vi "PCP return string to variant.vi"(1 "Action":T1, 7 "PCP return string":string, 11 "error in (no error)":errorcluster) -> (8 "Data":variant, 15 "error out":errorcluster)   [LabVIEW 2011]
uses:
  PCP Commands.ctl
  PCP return data types/RDd return.ctl
  PCP return data types/RA return Analog I.ctl
  PCP return data types/RP return digital IO.ctl
  PCP Command definer.ctl
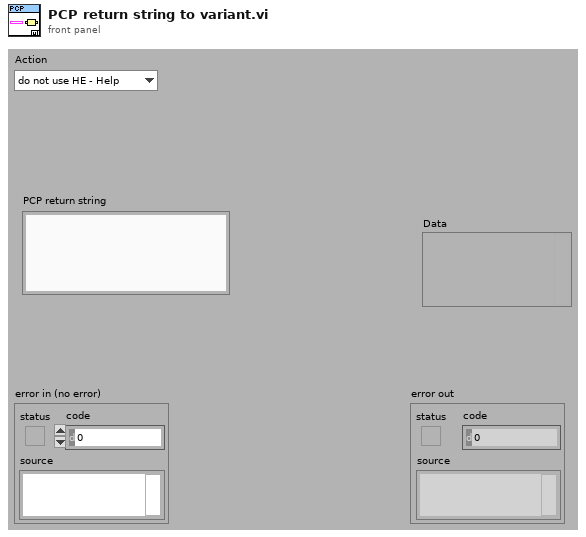
[diagram p1: front panel]
types:
  T1 = typedef "PCP Commands.ctl" = enum16{"do not use HE - Help", "RDd - Most used inputs", "RA - All analog inputs", "RE n Reset DO n", "SE n Set DO n", "RP - Get digital inputs", "VA d Set AO A  Motor Volt", "VB d Set AO B  Cable Resistance", "VEr - Get Version", "DYp - Depth counter", "DR - Reset Depth Counter", "DS n Set Depth options(0-3)", "do not use ME - Manual mode enabled", "MD - Manual mode disabled", "ID - Get ID(2001)", "TS - Get Timestamp", "TO d(s)  Set timeout", "do not use LO n Start Loop Mode(1,2)", "AL n RD&LO variation", "ST - Stop Loop Mode"}
  T2 = typedef "PCP Command definer.ctl" = cluster{"Action":T1, "n(0)":i32, "d(0.0)":dbl}
  T3 = typedef "RP return digital IO.ctl" = cluster{"DO -  HVPSU HV Off":bool, "DO -  HVPSU HV On":bool, "DI -  Unused 1":bool, "DO -  Local(T) / PC(F) mode":bool, "DI - Unused 2":bool, "DI - HVPSU HV On(T)":bool, "DI - PCP Local control(T)":bool, "DI - HVPSU On(T)":bool}
  T4 = typedef "RA return Analog I.ctl" = cluster{"HVPSU voltage output (AI 1)":dbl, "HVPSU current output (AI 2)":dbl, "PCP Motor voltage, head voltage (AI 3)":dbl, "PCP Cable resistance (AI 4)":dbl, "Cable tension (AI 5)":dbl, "CCL (AI 6)":dbl}
  T5 = typedef "RDd return.ctl" = cluster{"AI":T4, "Depth counter(Raw)":i32, "General Ratemeter":dbl, "Digital ports":T3}
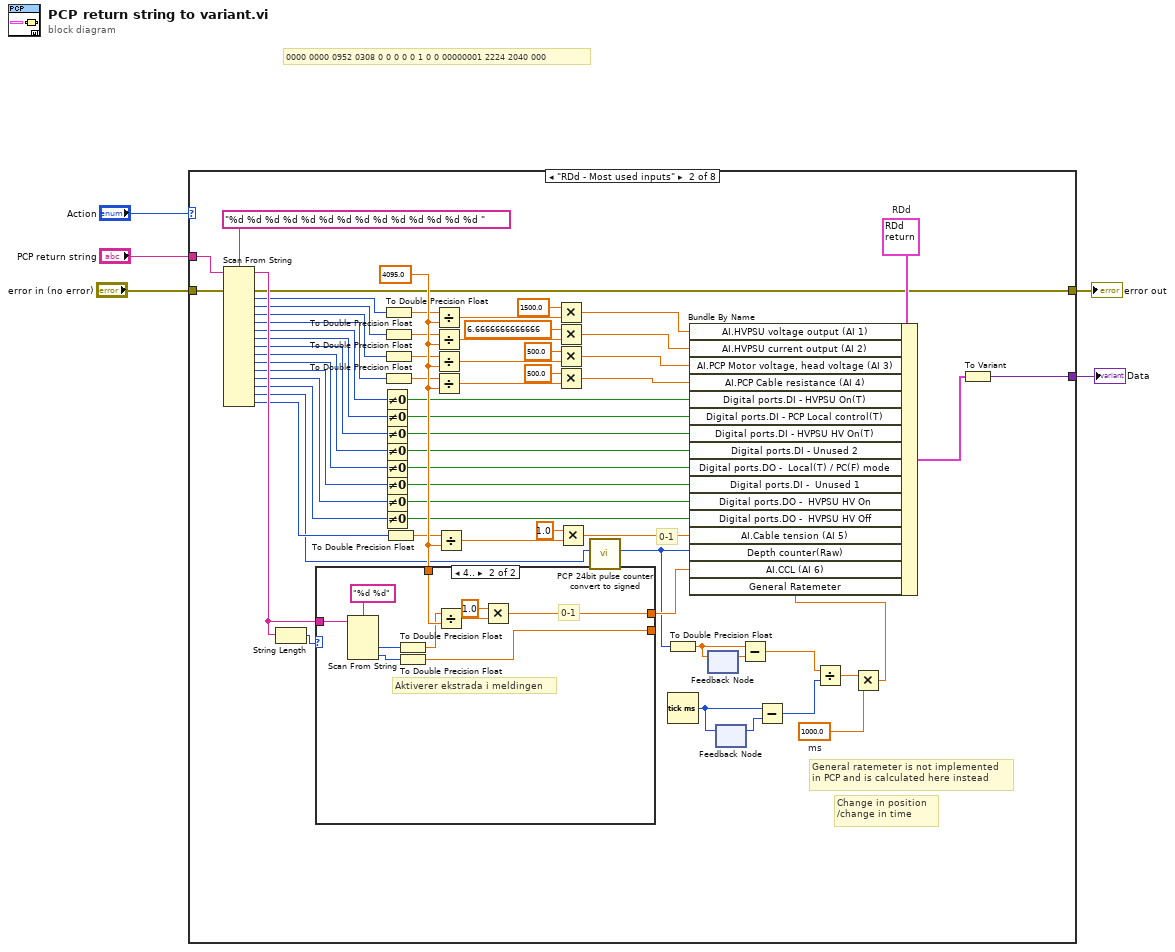
[diagram p0: block diagram]
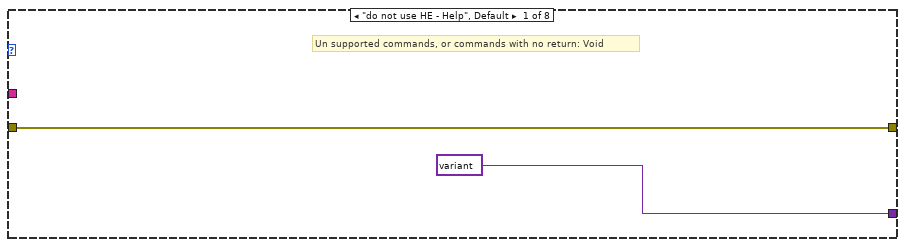
[diagram p2: hidden frame]
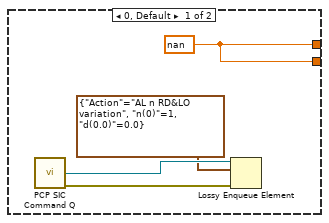
[diagram p3: hidden frame]
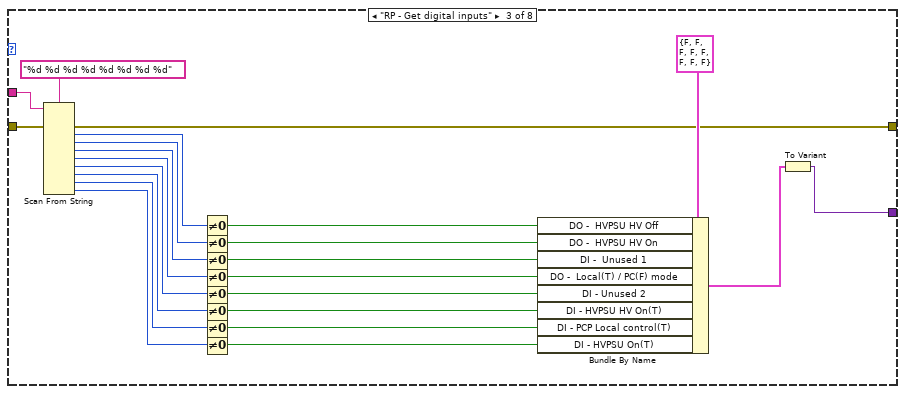
[diagram p4: hidden frame]
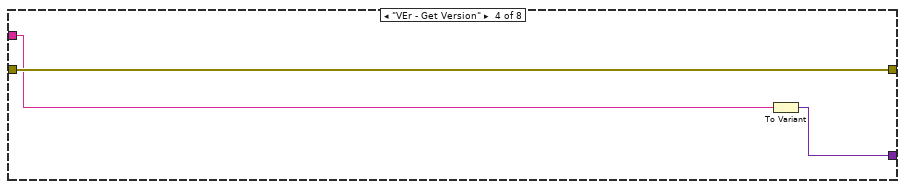
[diagram p5: hidden frame]
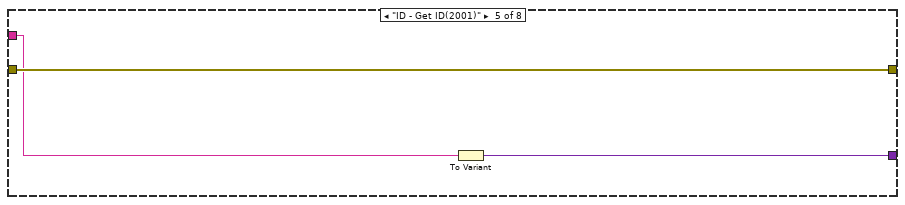
[diagram p6: hidden frame]
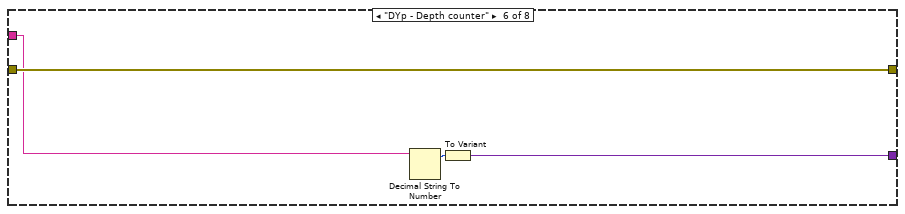
[diagram p7: hidden frame]
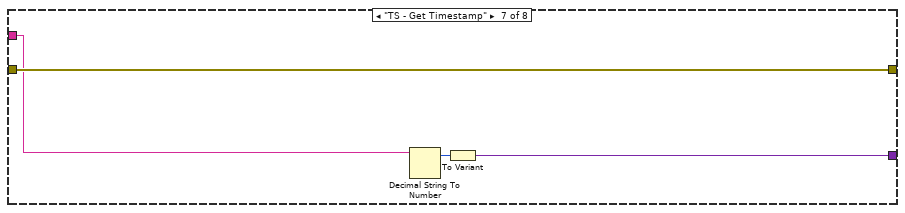
[diagram p8: hidden frame]
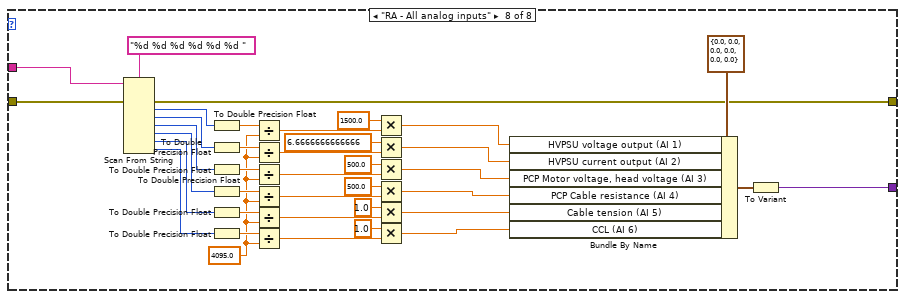
[diagram p9: hidden frame]
diagram:
  # "0000 0000 0952 0308 0 0 0 0 0 1 0 0 00000001 2224 2040 000"
  n1 = case shown="\"RDd - Most used inputs\"" "Action" {
    tunnel: [w7 w19 w85 w110 w113 w117 w121 w123] -> w4
    tunnel: "error in (no error)" -> [w7 w20 w86 w110 w113 w117 w121 w124]
    tunnel: "PCP return string" -> [_ w23 w91 w108 w111 w115 w119 w135]
    tunnel: [variant ("variant") w22 w90 w109 w112 w116 w120 w134] -> w1
    frame "do not use HE - Help", Default {
      # "Un supported commands, or commands with no return: Void"
    }
    frame "RDd - Most used inputs" {
      w9 = 1000.0  # ms
      w53 = T5 {"AI"={"HVPSU voltage output (AI 1)"=0.0, "HVPSU current output (AI 2)"=0.0, "PCP Motor voltage, head voltage (AI 3)"=0.0, "PCP Cable resistance (AI 4)"=0.0, "Cable tension (AI 5)"=0.0, "CCL (AI 6)"=0.0}, "Depth counter(Raw)"=0, "General Ratemeter"=0.0, "Digital ports"={"DO -  HVPSU HV Off"=FALSE, "DO -  HVPSU HV On"=FALSE, "DI -  Unused 1"=FALSE, "DO -  Local(T) / PC(F) mode"=FALSE, "DI - Unused 2"=FALSE, "DI - HVPSU HV On(T)"=FALSE, "DI - PCP Local control(T)"=FALSE, "DI - HVPSU On(T)"=FALSE}}  # RDd
      w70 = 4095.0 ("y")
      # "General ratemeter is not implemented\nin PCP and is calculated here instead"
      # "Change in position\n/change in time"
      # "0-1"
      n2 = Scan From String(format string="%d %d %d %d %d %d %d %d %d %d %d %d %d %d ", input string=w23, error in=w20) -> (remaining string=w69:string, error out=w19:errorcluster, output 1=w25:i32, output 2=w31:i32, output 3=w42:i32, output 4=w43:i32, output 5=w44:i32, output 6=w45:i32, output 7=w46:i32, output 8=w47:i32, output 9=w48:i32, output 10=w49:i32, output 11=w50:i32, output 12=w51:i32, output 13=w18:i32, output 14=w52:i32)  [unwired: 15 in, 1 out]
      n3 = String Length(string=w69) -> (length=w67:i32)
      n4 = case shown="4.." w67 {
        tunnel: [w74 w79] -> w68
        tunnel: [w74 w75] -> _
        tunnel: w69 -> [_ w83]
        tunnel: w70 -> [_ w80]
        frame 0, Default {
          w74 = nan
          n5 = call "PCP SIC Command Q.vi"() -> ("PCP cmd Q"=w72:refnum<queue>, "error out"=w73:errorcluster)  [unwired: 14 in]
          n6 = Lossy Enqueue Element(queue=w72, element=T2 {"Action"=enum."AL n RD&LO variation", "n(0)"=1, "d(0.0)"=0.0}, error in (no error)=w73) -> ()  [unwired: 4 out]
        }
        frame 4.. {
          # "Aktiverer ekstrada i meldingen"
          # "0-1"
          n7 = Scan From String(format string="%d %d", input string=w83) -> (output 1=w78:i32, output 2=w76:i32)  [unwired: 4 in, 3 out]
          n8 = To Double Precision Float(number=w78) -> (double precision float=w77:dbl)
          n9 = To Double Precision Float(number=w76) -> (double precision float=w75:dbl)
          n10 = Divide(x=w77, y=w80) -> (x/y=w82:dbl)
          n11 = Multiply(x=1.0, y=w82) -> (x*y=w79:dbl)
        }
      }
      n12 = Not Equal To 0?(x=w44) -> (x != 0?=w59:bool)
      n13 = Not Equal To 0?(x=w45) -> (x != 0?=w58:bool)
      n14 = Not Equal To 0?(x=w46) -> (x != 0?=w60:bool)
      n15 = Not Equal To 0?(x=w47) -> (x != 0?=w61:bool)
      n16 = Not Equal To 0?(x=w48) -> (x != 0?=w62:bool)
      n17 = Not Equal To 0?(x=w49) -> (x != 0?=w63:bool)
      n18 = Not Equal To 0?(x=w50) -> (x != 0?=w64:bool)
      n19 = Not Equal To 0?(x=w51) -> (x != 0?=w65:bool)
      n20 = To Double Precision Float(number=w25) -> (double precision float=w26:dbl)
      n21 = To Double Precision Float(number=w31) -> (double precision float=w30:dbl)
      n22 = To Double Precision Float(number=w42) -> (double precision float=w34:dbl)
      n23 = To Double Precision Float(number=w43) -> (double precision float=w37:dbl)
      n24 = To Double Precision Float(number=w52) -> (double precision float=w40:dbl)
      n25 = Divide(x=w26, y=w70) -> (x/y=w27:dbl)
      n26 = Divide(x=w30, y=w70) -> (x/y=w29:dbl)
      n27 = Divide(x=w34, y=w70) -> (x/y=w35:dbl)
      n28 = Divide(x=w37, y=w70) -> (x/y=w36:dbl)
      n29 = Divide(x=w40, y=w70) -> (x/y=w41:dbl)
      n30 = Multiply(x=1500.0, y=w27) -> (x*y=w54:dbl)
      n31 = Multiply(x=6.6666666666666, y=w29) -> (x*y=w55:dbl)
      n32 = Multiply(x=500.0, y=w35) -> (x*y=w56:dbl)
      n33 = Multiply(x=500.0, y=w36) -> (x*y=w57:dbl)
      n34 = Multiply(x=1.0, y=w41) -> (x*y=w66:dbl)
      n35 = call "PCP 24bit pulse counter convert to signed.vi"("24 bit puls counter input"=w18) -> ("signed pulse counter output"=w17:i32)  [unwired: 10 in]
      n36 = To Double Precision Float(number=w17) -> (double precision float=w16:dbl)
      n37 = Tick Count (ms)() -> (millisecond timer value=w14:u32)
      n38 = feedback-in #1(w16) -> ()
      n39 = feedback #1() -> (w15:dbl)  [unwired: 1 in]
      n40 = feedback #2() -> (w13:u32)  [unwired: 1 in]
      n41 = feedback-in #2(w14) -> ()
      n42 = Subtract(x=w16, y=w15) -> (x-y=w12:dbl)
      n43 = Subtract(x=w14, y=w13) -> (x-y=w11:u32)
      n44 = Divide(x=w12, y=w11) -> (x/y=w10:dbl)
      n45 = Multiply(x=w10, y=w9) -> (x*y=w8:dbl)
      n46 = Bundle By Name(cluster=w53, "AI.HVPSU voltage output (AI 1)"=w54, "AI.HVPSU current output (AI 2)"=w55, "AI.PCP Motor voltage, head voltage (AI 3)"=w56, "AI.PCP Cable resistance (AI 4)"=w57, "Digital ports.DI - HVPSU On(T)"=w59, "Digital ports.DI - PCP Local control(T)"=w58, "Digital ports.DI - HVPSU HV On(T)"=w60, "Digital ports.DI - Unused 2"=w61, "Digital ports.DO -  Local(T) / PC(F) mode"=w62, "Digital ports.DI -  Unused 1"=w63, "Digital ports.DO -  HVPSU HV On"=w64, "Digital ports.DO -  HVPSU HV Off"=w65, "AI.Cable tension (AI 5)"=w66, "Depth counter(Raw)"=w17, "AI.CCL (AI 6)"=w68, "General Ratemeter"=w8) -> (w21:T5)
      n47 = To Variant(anything=w21) -> (Variant=w22:variant)
    }
    frame "RP - Get digital inputs" {
      n48 = Scan From String(format string="%d %d %d %d %d %d %d %d", input string=w91, error in=w86) -> (error out=w85:errorcluster, output 1=w92:i32, output 2=w93:i32, output 3=w94:i32, output 4=w95:i32, output 5=w96:i32, output 6=w97:i32, output 7=w98:i32, output 8=w99:i32)  [unwired: 9 in, 2 out]
      n49 = Not Equal To 0?(x=w92) -> (x != 0?=w101:bool)
      n50 = Not Equal To 0?(x=w93) -> (x != 0?=w100:bool)
      n51 = Not Equal To 0?(x=w94) -> (x != 0?=w102:bool)
      n52 = Not Equal To 0?(x=w95) -> (x != 0?=w103:bool)
      n53 = Not Equal To 0?(x=w96) -> (x != 0?=w104:bool)
      n54 = Not Equal To 0?(x=w97) -> (x != 0?=w105:bool)
      n55 = Not Equal To 0?(x=w98) -> (x != 0?=w106:bool)
      n56 = Not Equal To 0?(x=w99) -> (x != 0?=w107:bool)
      n57 = Bundle By Name(cluster=T3 {"DO -  HVPSU HV Off"=FALSE, "DO -  HVPSU HV On"=FALSE, "DI -  Unused 1"=FALSE, "DO -  Local(T) / PC(F) mode"=FALSE, "DI - Unused 2"=FALSE, "DI - HVPSU HV On(T)"=FALSE, "DI - PCP Local control(T)"=FALSE, "DI - HVPSU On(T)"=FALSE} ("Digital ports"), "DO -  HVPSU HV Off"=w101, "DO -  HVPSU HV On"=w100, "DI -  Unused 1"=w102, "DO -  Local(T) / PC(F) mode"=w103, "DI - Unused 2"=w104, "DI - HVPSU HV On(T)"=w105, "DI - PCP Local control(T)"=w106, "DI - HVPSU On(T)"=w107) -> (w89:T3)
      n58 = To Variant(anything=w89) -> (Variant=w90:variant)
    }
    frame "VEr - Get Version" {
      n59 = To Variant(anything=w108) -> (Variant=w109:variant)
    }
    frame "ID - Get ID(2001)" {
      n60 = To Variant(anything=w111) -> (Variant=w112:variant)
    }
    frame "DYp - Depth counter" {
      n61 = Decimal String To Number(string=w115) -> (offset past number=w114:i32)  [unwired: 2 in, 1 out]
      n62 = To Variant(anything=w114) -> (Variant=w116:variant)
    }
    frame "TS - Get Timestamp" {
      n63 = Decimal String To Number(string=w119) -> (offset past number=w118:i32)  [unwired: 2 in, 1 out]
      n64 = To Variant(anything=w118) -> (Variant=w120:variant)
    }
    frame "RA - All analog inputs" {
      w122 = 4095.0 ("y")
      n65 = Scan From String(format string="%d %d %d %d %d %d ", input string=w135, error in=w124) -> (error out=w123:errorcluster, output 1=w137:i32, output 2=w143:i32, output 3=w154:i32, output 4=w155:i32, output 5=w130:i32, output 6=w126:i32)  [unwired: 7 in, 2 out]
      n66 = To Double Precision Float(number=w137) -> (double precision float=w138:dbl)
      n67 = To Double Precision Float(number=w143) -> (double precision float=w142:dbl)
      n68 = To Double Precision Float(number=w154) -> (double precision float=w146:dbl)
      n69 = To Double Precision Float(number=w155) -> (double precision float=w149:dbl)
      n70 = To Double Precision Float(number=w130) -> (double precision float=w152:dbl)
      n71 = To Double Precision Float(number=w126) -> (double precision float=w129:dbl)
      n72 = Divide(x=w138, y=w122) -> (x/y=w139:dbl)
      n73 = Divide(x=w142, y=w122) -> (x/y=w141:dbl)
      n74 = Divide(x=w146, y=w122) -> (x/y=w147:dbl)
      n75 = Divide(x=w149, y=w122) -> (x/y=w148:dbl)
      n76 = Divide(x=w152, y=w122) -> (x/y=w153:dbl)
      n77 = Divide(x=w129, y=w122) -> (x/y=w128:dbl)
      n78 = Multiply(x=1500.0, y=w139) -> (x*y=w156:dbl)
      n79 = Multiply(x=6.6666666666666, y=w141) -> (x*y=w157:dbl)
      n80 = Multiply(x=500.0, y=w147) -> (x*y=w158:dbl)
      n81 = Multiply(x=500.0, y=w148) -> (x*y=w159:dbl)
      n82 = Multiply(x=1.0, y=w153) -> (x*y=w131:dbl)
      n83 = Multiply(x=1.0, y=w128) -> (x*y=w125:dbl)
      n84 = Bundle By Name(cluster=T4 {"HVPSU voltage output (AI 1)"=0.0, "HVPSU current output (AI 2)"=0.0, "PCP Motor voltage, head voltage (AI 3)"=0.0, "PCP Cable resistance (AI 4)"=0.0, "Cable tension (AI 5)"=0.0, "CCL (AI 6)"=0.0} ("AI"), "HVPSU voltage output (AI 1)"=w156, "HVPSU current output (AI 2)"=w157, "PCP Motor voltage, head voltage (AI 3)"=w158, "PCP Cable resistance (AI 4)"=w159, "Cable tension (AI 5)"=w131, "CCL (AI 6)"=w125) -> (w133:T4)
      n85 = To Variant(anything=w133) -> (Variant=w134:variant)
    }
  }
  "error out" <- w4
  "Data" <- w1
